vi "MGCC_ProtCoord_main.vi"   [LabVIEW 2016]
uses:
  <vilib>/imath/engines/lvmath2/RunTimeEngine/VariableToken/NIMS_VariableToken_CondDefined.vi
  <instcachedir>/0/NIMS_VariableToken_CondDefined_06E9DA95BD4D46A6BA55EC651A891960.lvgen/NIMS_VariableToken_CondDefined_06E9DA95BD4D46A6BA55EC651A891960_006.vi
  <vilib>/imathl/engines/lvmath/Functions/Error Handling/Create Error.vi
  <vilib>/imath/engines/lvmath2/RunTimeEngine/NodeEndStatement/NIMS_NodeEndStatement_Output.vi
  <instcachedir>/0/NIMS_NodeEndStatement_Output_53EC0D466D134D7ABD903AC30B43404B.lvgen/NIMS_NodeEndStatement_Output_53EC0D466D134D7ABD903AC30B43404B_011.vi
  <vilib>/imath/engines/lvmath2/RunTimeEngine/ErrorHandling/NIMS_Finalize Error.vi
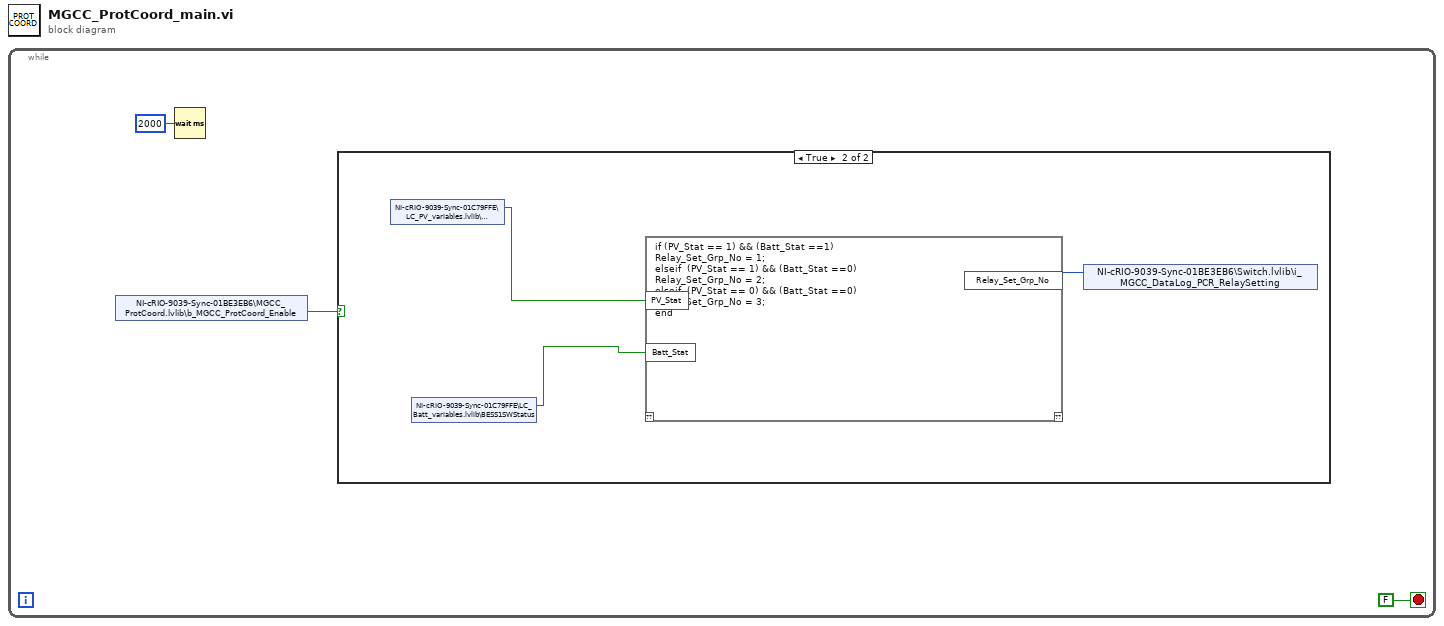
[diagram p0: block diagram]
diagram:
  n1 = while {
    stop <- FALSE stop-if-true
    n2 = shared-variable "NI-cRIO-9039-Sync-01BE3EB6\\MGCC_ProtCoord.lvlib\\b_MGCC_ProtCoord_Enable"() -> (w3:bool)  [unwired: 1 in, 1 out]
    n3 = Wait (ms)(milliseconds to wait=u32 2000) -> ()  [unwired: 1 out]
    n4 = case shown="True" w3 {
      frame False {
      }
      frame True {
        n5 = shared-variable "NI-cRIO-9039-Sync-01C79FFE\\LC_PV_variables.lvlib\\PV1SWStatus"() -> (w5:bool)  [unwired: 1 in, 1 out]
        n6 = shared-variable "NI-cRIO-9039-Sync-01C79FFE\\LC_Batt_variables.lvlib\\BESS1SWStatus"() -> (w4:bool)  [unwired: 1 in, 1 out]
        n7 = mathscript code="if (PV_Stat == 1) && (Batt_Stat ==1)\nRelay_Set_Grp_No = 1;\nelseif  (PV_Stat == 1) && (Batt_Stat ==0)\nRelay_Set_Grp_No = 2;\nelseif  (PV_Stat == 0) && (Batt_Stat ==0)\nRelay_Set_Grp_No = 3;\nend"("PV_Stat"=w5, "Batt_Stat"=w4) -> ("Relay_Set_Grp_No"=w6:i32)  [unwired: 1 in, 1 out]
        n8 = shared-variable "NI-cRIO-9039-Sync-01BE3EB6\\Switch.lvlib\\i_MGCC_DataLog_PCR_RelaySetting"(w6) -> ()  [unwired: 1 in, 1 out]
      }
    }
  }
